vi "test Fails If Arrays Are Not Equal With Multiple Failures.vi"(8 "error in (no error)":errorcluster, 11 "TestCase in":refnum<class "Pass If Equal 1D Array (String) Test Case.lvclass">) -> (0 "error out":errorcluster, 3 "TestCase out":refnum<class "Pass If Equal 1D Array (String) Test Case.lvclass">)   [LabVIEW 2015, in "Pass If Equal 1D Array (String) Test Case.lvclass"]
uses:
  Pass If Equal 1D Array (String) Test Case.lvclass
  <vilib>/addons/_JKI Toolkits/VI Tester/TestCase.llb/TestCase.lvclass
  VITAC.lvlib
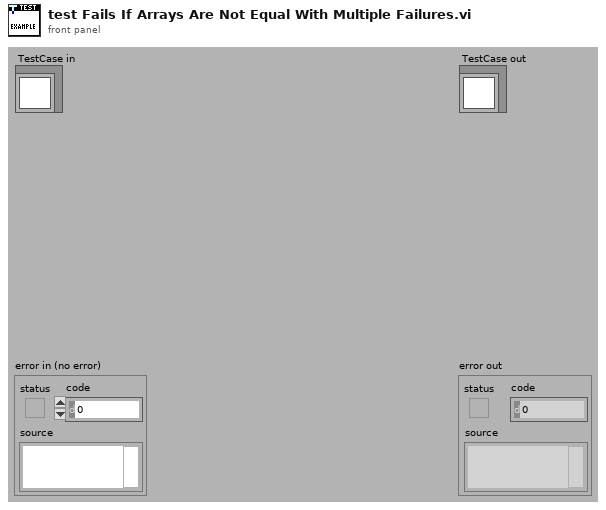
[diagram p1: front panel]
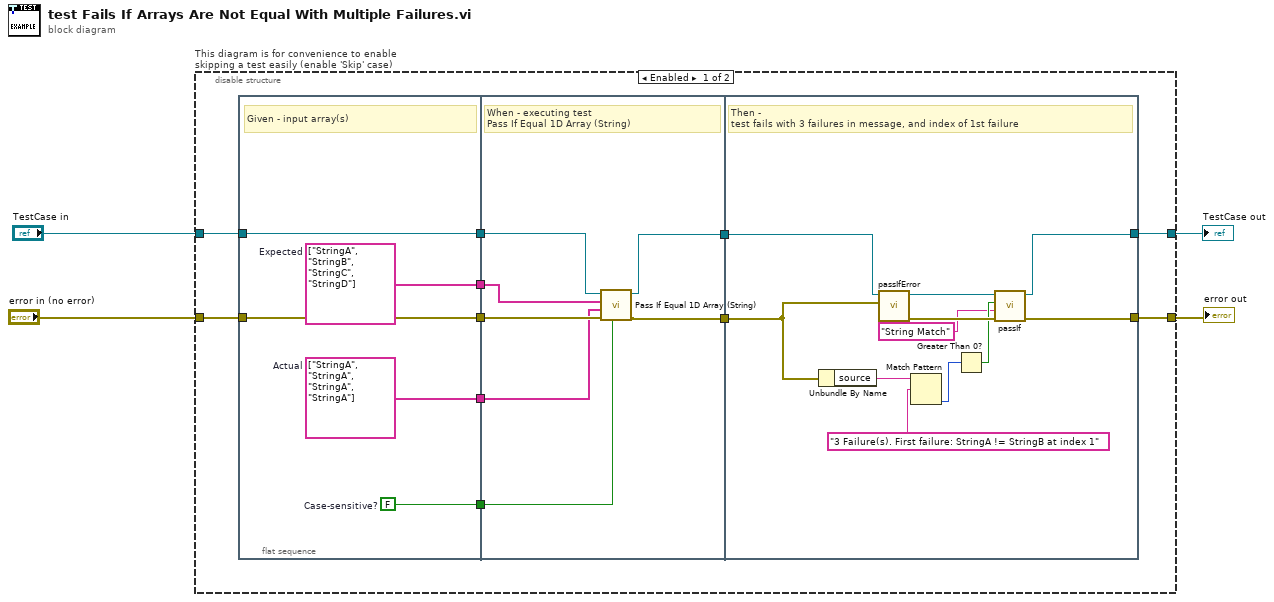
[diagram p0: block diagram]
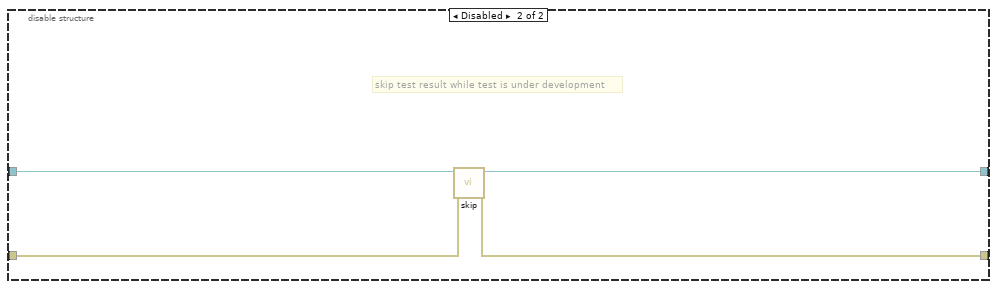
[diagram p2: hidden frame]
diagram:
  n1 = disable-structure "This diagram is for convenience to enable skipping a test easily (enable 'Skip' case)" shown="Enabled" {
    disable-tunnel: "TestCase in" -> [w13 w42]
    disable-tunnel: [w15 w40] -> w1
    disable-tunnel: [w12 w41] -> w3
    disable-tunnel: "error in (no error)" -> [w10 w39]
    frame Enabled {
      n2 = flat-sequence {
        tunnel: [w20] -> w14
        tunnel: w13 -> [w20]
        tunnel: [w19] -> w11
        tunnel: w10 -> [w19]
        tunnel: [w18] -> w9
        tunnel: [w17] -> w8
        tunnel: [w16] -> w7
        tunnel: w14 -> [w26]
        tunnel: w11 -> [w27]
        tunnel: w9 -> [w25]
        tunnel: w8 -> [w24]
        tunnel: w7 -> [w23]
        tunnel: [w22] -> w6
        tunnel: [w21] -> w5
        tunnel: [w30] -> w15
        tunnel: [w31] -> w12
        tunnel: w6 -> [w29]
        tunnel: w5 -> [w28]
        frame #0 {
          w18 = FALSE  # Case-sensitive?
          w17 = string[] ["StringA", "StringA", "StringA", "StringA"]  # Actual
          w16 = string[] ["StringA", "StringB", "StringC", "StringD"]  # Expected
          # "Given - input array(s)"
        }
        frame #1 {
          # "When - executing test \nPass If Equal 1D Array (String)"
          n3 = call "Pass If Equal 1D Array (String).vi"("case sensitive?"=w25, "error in (no error)"=w27, "actual"=w24, "expected"=w23, "TestCase in"=w26) -> ("error out"=w21:errorcluster, "TestCase out"=w22:refnum<class "Pass If Equal 1D Array (String) Test Case.lvclass">)  [unwired: 5 in]
        }
        frame #2 {
          # "Then - \ntest fails with 3 failures in message, and index of 1st failure"
          n4 = Unbundle By Name(w28) -> ("source"=w36:string)
          n5 = call-dynamic "passIfError.vi"("error"=w28, "TestCase in"=w29) -> ("error out"=w38:errorcluster, "TestCase out"=w37:refnum<class "Pass If Equal 1D Array (String) Test Case.lvclass">)  [unwired: 8 in]
          n6 = Match Pattern(string=w36, regular expression="3 Failure(s). First failure: StringA != StringB at index 1") -> (offset past match=w34:i32)  [unwired: 1 in, 3 out]
          n7 = Greater Than 0?(x=w34) -> (x > 0?=w33:bool)
          n8 = call-dynamic "passIf.vi"("error in (no error)"=w38, "message (\"\")"="String Match" ("message (\"\")"), "pass"=w33, "TestCase in"=w37) -> ("error out"=w31:errorcluster, "TestCase out"=w30:refnum<class "Pass If Equal 1D Array (String) Test Case.lvclass">)  [unwired: 6 in]
        }
      }
    }
    frame Disabled {
      # "skip test result while test is under development"
      n9 = call <vilib>:"skip.vi"("error in (no error)"=w39, "TestCase in"=w42) -> ("error out"=w41:errorcluster, "TestCase out"=w40:refnum<class "Pass If Equal 1D Array (String) Test Case.lvclass">)  [unwired: 8 in]
    }
  }
  "error out" <- w3
  "TestCase out" <- w1
